vi "ProcessCameraImages.vi"(1 "Margin of Error":i32=10, 5 "Blue or Luma or Val or Inten Range":cluster{"Lower value":i32, "Upper value":i32}={"Lower value"=20, "Upper value"=120}, 6 "Green or Sat Range":cluster{"Lower value":i32, "Upper value":i32}={"Lower value"=0, "Upper value"=255}, 7 "Red or Hue Range":cluster{"Lower value":i32, "Upper value":i32}={"Lower value"=80, "Upper value"=100}, 8 "Draw Targets":bool, 9 "R_Image":T2, 10 "L_Image":T2) -> (0 "Procesing Time":u32, 2 "TargetMatch":T1(array[cluster]), 3 "L_Image Out":T2, 4 "R_Image Out":T2)   [LabVIEW 2011]
uses:
  <vilib>/vision/Image Controls.llb/IMAQ Image.ctl
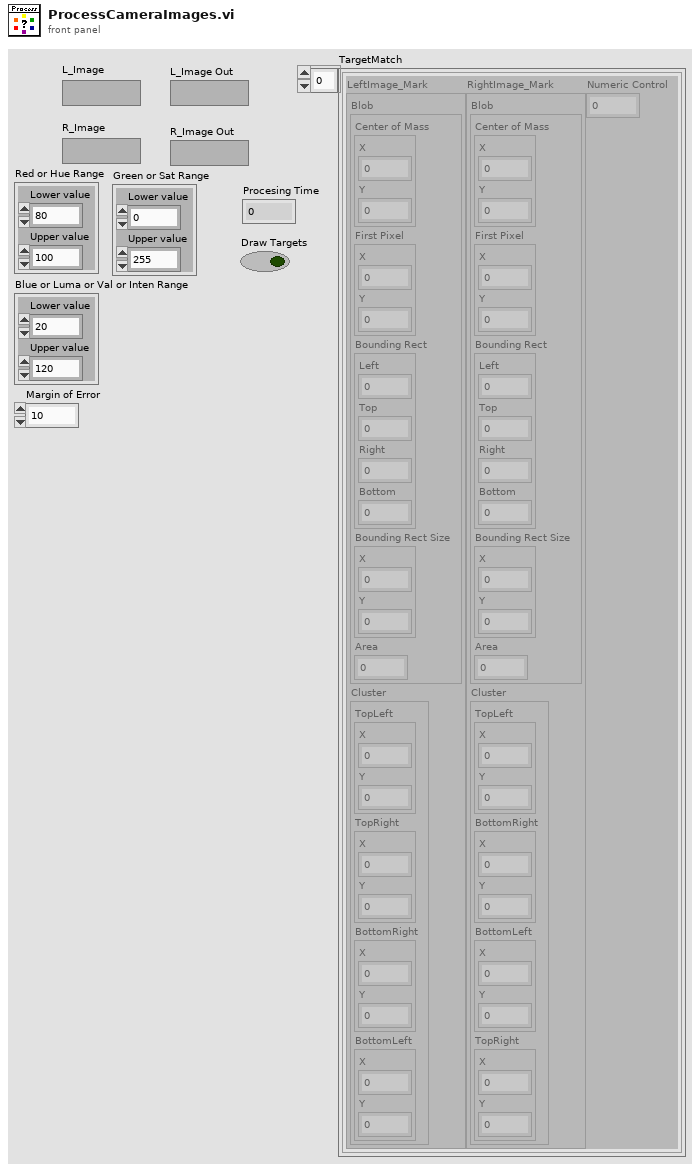
[diagram p1: front panel]
types:
  T1 = cluster{"LeftImage_Mark":cluster{"Blob":cluster{"Center of Mass":cluster{"X":dbl, "Y":dbl}, "First Pixel":cluster{"X":dbl, "Y":dbl}, "Bounding Rect":cluster{"Left":dbl, "Top":dbl, "Right":dbl, "Bottom":dbl}, "Bounding Rect Size":cluster{"X":dbl, "Y":dbl}, "Area":dbl}, "Cluster":cluster{"TopLeft":cluster{"X":dbl, "Y":dbl}, "TopRight":cluster{"X":dbl, "Y":dbl}, "BottomRight":cluster{"X":dbl, "Y":dbl}, "BottomLeft":cluster{"X":dbl, "Y":dbl}}}, "RightImage_Mark":cluster{"Blob":cluster{"Center of Mass":cluster{"X":dbl, "Y":dbl}, "First Pixel":cluster{"X":dbl, "Y":dbl}, "Bounding Rect":cluster{"Left":dbl, "Top":dbl, "Right":dbl, "Bottom":dbl}, "Bounding Rect Size":cluster{"X":dbl, "Y":dbl}, "Area":dbl}, "Cluster":cluster{"TopLeft":cluster{"X":dbl, "Y":dbl}, "BottomRight":cluster{"X":dbl, "Y":dbl}, "BottomLeft":cluster{"X":dbl, "Y":dbl}, "TopRight":cluster{"X":dbl, "Y":dbl}}}, "Numeric Control":dbl}[]
  T2 = typedef "IMAQ Image.ctl" = refnum<image>
  T3 = typedef "Image Type" = u32
  T4 = cluster{"Center of Mass":cluster{"X":dbl, "Y":dbl}, "First Pixel":cluster{"X":dbl, "Y":dbl}, "Bounding Rect":cluster{"Left":dbl, "Top":dbl, "Right":dbl, "Bottom":dbl}, "Bounding Rect Size":cluster{"X":dbl, "Y":dbl}, "Area":dbl}[]
  T5 = cluster{"Start Point":cluster{"X":sgl, "Y":sgl}, "End Point":cluster{"X":sgl, "Y":sgl}, "Length":dbl, "Orientation":dbl, "Score":dbl}[]
  T6 = cluster{"Blob":cluster{"Center of Mass":cluster{"X":dbl, "Y":dbl}, "First Pixel":cluster{"X":dbl, "Y":dbl}, "Bounding Rect":cluster{"Left":dbl, "Top":dbl, "Right":dbl, "Bottom":dbl}, "Bounding Rect Size":cluster{"X":dbl, "Y":dbl}, "Area":dbl}, "Corners":cluster{"TopLeft":cluster{"X":dbl, "Y":dbl}, "TopRight":cluster{"X":dbl, "Y":dbl}, "BottomRight":cluster{"X":dbl, "Y":dbl}, "BottomLeft":cluster{"X":dbl, "Y":dbl}}}[]
  T7 = cluster{"LeftImage_Mark":cluster{"Blob":cluster{"Center of Mass":cluster{"X":dbl, "Y":dbl}, "First Pixel":cluster{"X":dbl, "Y":dbl}, "Bounding Rect":cluster{"Left":dbl, "Top":dbl, "Right":dbl, "Bottom":dbl}, "Bounding Rect Size":cluster{"X":dbl, "Y":dbl}, "Area":dbl}, "Corners":cluster{"TopLeft":cluster{"X":dbl, "Y":dbl}, "TopRight":cluster{"X":dbl, "Y":dbl}, "BottomRight":cluster{"X":dbl, "Y":dbl}, "BottomLeft":cluster{"X":dbl, "Y":dbl}}}, "RightImage_Mark":cluster{"Blob":cluster{"Center of Mass":cluster{"X":dbl, "Y":dbl}, "First Pixel":cluster{"X":dbl, "Y":dbl}, "Bounding Rect":cluster{"Left":dbl, "Top":dbl, "Right":dbl, "Bottom":dbl}, "Bounding Rect Size":cluster{"X":dbl, "Y":dbl}, "Area":dbl}, "Corners":cluster{"TopLeft":cluster{"X":dbl, "Y":dbl}, "BottomRight":cluster{"X":dbl, "Y":dbl}, "BottomLeft":cluster{"X":dbl, "Y":dbl}, "TopRight":cluster{"X":dbl, "Y":dbl}}}, "Score":dbl}[]
  T8 = cluster{"Blob":cluster{"Center of Mass":cluster{"X":dbl, "Y":dbl}, "First Pixel":cluster{"X":dbl, "Y":dbl}, "Bounding Rect":cluster{"Left":dbl, "Top":dbl, "Right":dbl, "Bottom":dbl}, "Bounding Rect Size":cluster{"X":dbl, "Y":dbl}, "Area":dbl}, "Corners":cluster{"TopLeft":cluster{"X":dbl, "Y":dbl}, "TopRight":cluster{"X":dbl, "Y":dbl}, "BottomRight":cluster{"X":dbl, "Y":dbl}, "BottomLeft":cluster{"X":dbl, "Y":dbl}}}
  T9 = cluster{"Blob":cluster{"Center of Mass":cluster{"X":dbl, "Y":dbl}, "First Pixel":cluster{"X":dbl, "Y":dbl}, "Bounding Rect":cluster{"Left":dbl, "Top":dbl, "Right":dbl, "Bottom":dbl}, "Bounding Rect Size":cluster{"X":dbl, "Y":dbl}, "Area":dbl}, "Corners":cluster{"TopLeft":cluster{"X":dbl, "Y":dbl}, "BottomRight":cluster{"X":dbl, "Y":dbl}, "BottomLeft":cluster{"X":dbl, "Y":dbl}, "TopRight":cluster{"X":dbl, "Y":dbl}}}
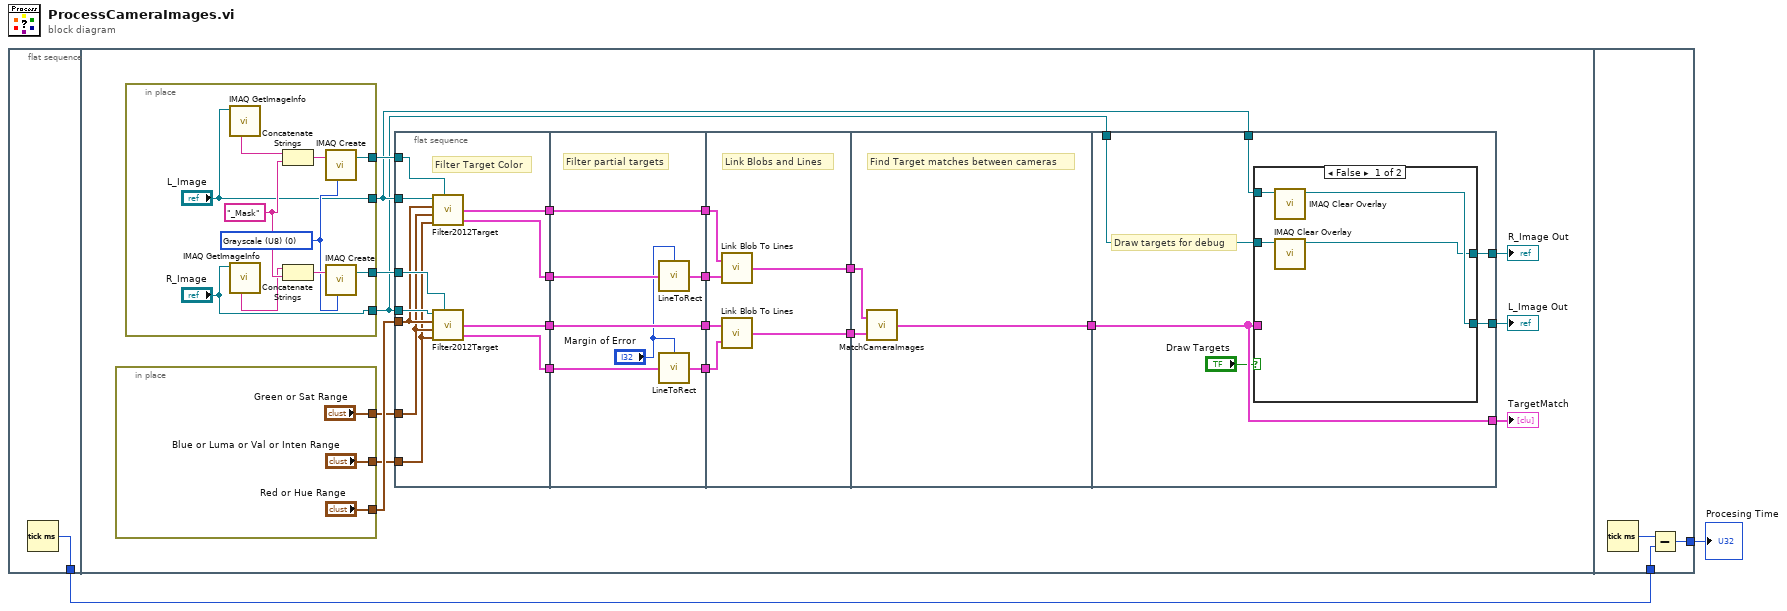
[diagram p0: block diagram]
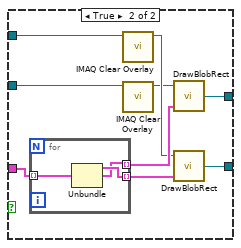
[diagram p2: hidden frame]
diagram:
  n1 = flat-sequence {
    tunnel: [w3] -> w2
    tunnel: w2 -> [w88]
    tunnel: [w87] -> w1
    frame #0 {
      n2 = Tick Count (ms)() -> (millisecond timer value=w3:u32)
    }
    frame #1 {
      n3 = in-place {
        in-place-border: ["Red or Hue Range"] -> w6
        in-place-border: ["Blue or Luma or Val or Inten Range"] -> w4
        in-place-border: ["Green or Sat Range"] -> w5
      }
      n4 = in-place {
        in-place-border: [w34] -> w21
        in-place-border: [w30] -> w20
        in-place-border: ["L_Image"] -> w19
        in-place-border: ["R_Image"] -> w18
        w27 = T3 0 items=["Grayscale (U8)", "Grayscale (I16)", "Grayscale (SGL)", "Complex (CSG)", "RGB (U32)", "HSL (U32)", "RGB (U64)", "Grayscale (U16)"] ("Image Type")
        w29 = "_Mask" ("string")
        n5 = call "IMAQ GetImageInfo"("Image"="L_Image") -> ("Image Name"=w32:string)  [unwired: 3 in, 7 out]
        n6 = call "IMAQ GetImageInfo"("Image"="R_Image") -> ("Image Name"=w28:string)  [unwired: 3 in, 7 out]
        n7 = Concatenate Strings(w32, w29) -> (w33:string)
        n8 = Concatenate Strings(w28, w29) -> (w31:string)
        n9 = call "IMAQ Create"("Image Name"=w33, "Image Type"=w27) -> ("New Image"=w34:T2)  [unwired: 3 in, 1 out]
        n10 = call "IMAQ Create"("Image Name"=w31, "Image Type"=w27) -> ("New Image"=w30:T2)  [unwired: 3 in, 1 out]
      }
      n11 = flat-sequence {
        tunnel: w18 -> [w45]
        tunnel: w19 -> [w46]
        tunnel: w21 -> [w48]
        tunnel: w20 -> [w47]
        tunnel: [w44] -> w13
        tunnel: [w43] -> w10
        tunnel: [w42] -> w8
        tunnel: [w41] -> w7
        tunnel: w6 -> [w40]
        tunnel: w5 -> [w39]
        tunnel: w4 -> [w38]
        tunnel: [w49] -> w14
        tunnel: w13 -> [w55]
        tunnel: [w55] -> w12
        tunnel: [w52] -> w11
        tunnel: w10 -> [w54]
        tunnel: [w54] -> w9
        tunnel: w8 -> [w51]
        tunnel: w7 -> [w53]
        tunnel: [w61] -> w24
        tunnel: [w60] -> w23
        tunnel: w14 -> [w56]
        tunnel: w12 -> [w57]
        tunnel: w11 -> [w58]
        tunnel: w9 -> [w59]
        tunnel: w24 -> [w63]
        tunnel: w23 -> [w64]
        tunnel: [w62] -> w22
        tunnel: w19 -> [w70]
        tunnel: w18 -> [w69]
        tunnel: [w68] -> w17
        tunnel: [w67] -> w16
        tunnel: [w66] -> w15
        tunnel: w22 -> [w66]
        frame #0 {
          # "Filter Target Color"
          n12 = call "Filter2012Target.vi"("Image In"=w46, "Red or Hue Range"=w40, "Green or Sat Range"=w39, "Blue or Luma or Val or Inten Range"=w38, "Image Dst"=w48) -> ("Blob Array"=w44:T4, "Lines Calibrated"=w42:T5)  [unwired: 1 out]
          n13 = call "Filter2012Target.vi"("Image In"=w45, "Red or Hue Range"=w40, "Green or Sat Range"=w39, "Blue or Luma or Val or Inten Range"=w38, "Image Dst"=w47) -> ("Blob Array"=w43:T4, "Lines Calibrated"=w41:T5)  [unwired: 1 out]
        }
        frame #1 {
          # "Filter partial targets"
          n14 = call "LineToRect.vi"("Lines"=w51, "Margin of Error"="Margin of Error") -> ("Good Lines"=w49:T5)
          n15 = call "LineToRect.vi"("Lines"=w53, "Margin of Error"="Margin of Error") -> ("Good Lines"=w52:T5)
        }
        frame #2 {
          # "Link Blobs and Lines"
          n16 = call "Link Blob To Lines.vi"("Lines Calibrated"=w56, "Blob Array"=w57) -> ("TargetArray"=w60:T6)
          n17 = call "Link Blob To Lines.vi"("Lines Calibrated"=w58, "Blob Array"=w59) -> ("TargetArray"=w61:T6)
        }
        frame #3 {
          # "Find Target matches between cameras"
          n18 = call "MatchCameraImages.vi"("R_TargetArray"=w63, "L_TargetArray"=w64) -> ("TargetMatch"=w62:T7)
        }
        frame #4 {
          # "Draw targets for debug"
          n19 = case shown="False" "Draw Targets" {
            tunnel: w70 -> [w74 w83]
            tunnel: w69 -> [w72 w82]
            tunnel: [w73 w79] -> w68
            tunnel: [w71 w78] -> w67
            tunnel: w66 -> [_ w77]
            frame False {
              n20 = call "IMAQ Clear Overlay"("Image"=w74) -> ("Image Out"=w73:T2)  [unwired: 9 in, 1 out]
              n21 = call "IMAQ Clear Overlay"("Image"=w72) -> ("Image Out"=w71:T2)  [unwired: 9 in, 1 out]
            }
            frame True {
              n22 = for {
                tunnel: w77 -> [w86] mode=indexing
                tunnel: [w85] -> w80 mode=indexing
                tunnel: [w84] -> w81 mode=indexing
                n23 = Unbundle(w86) -> ("LeftImage_Mark"=w85:T8, "RightImage_Mark"=w84:T9)  [unwired: 1 out]
              }
              n24 = call "IMAQ Clear Overlay"("Image"=w83) -> ("Image Out"=w76:T2)  [unwired: 9 in, 1 out]
              n25 = call "IMAQ Clear Overlay"("Image"=w82) -> ("Image Out"=w75:T2)  [unwired: 9 in, 1 out]
              n26 = call "DrawBlobRect.vi"("BlobLineDataArray"=w81, "Src In"=w75) -> ("Image Out"=w78:T2)  [unwired: 1 in]
              n27 = call "DrawBlobRect.vi"("BlobLineDataArray"=w80, "Src In"=w76) -> ("Image Out"=w79:T2)  [unwired: 1 in]
            }
          }
        }
      }
      "L_Image Out" <- w17
      "R_Image Out" <- w16
      "TargetMatch" <- w15
    }
    frame #2 {
      n28 = Tick Count (ms)() -> (millisecond timer value=w89:u32)
      n29 = Subtract(x=w89, y=w88) -> (x-y=w87:u32)
    }
  }
  "Procesing Time" <- w1
